vi "students-estimator.vi"() -> (0 "Estimator Script Error":errorcluster, 1 "Estimator State Space Object":T2 {"Transport Delay" format="%.2f"; "D" format="%#.2g"; "C" format="%#.2g"; "B" format="%#.2g"; "A" format="%#.2g"; "properties"."Sampling Time" format="%#.6p"; "properties"."Output Delays" format="%.4f"; "properties"."Input Delays" format="%.4f"}, 2 "State Feedback Gain (K)":T1, 3 "Input Scaling (Nbar)":dbl)   [LabVIEW 2009]
uses:
  <vilib>/addons/Control Design/_Model Construction/Model Typedefs.llb/CD State Space Model (MIMO).ctl
  <vilib>/addons/Control Design/_Model Construction/Model Typedefs.llb/CD General Elements.ctl
  <vilib>/Analysis/Matrix/Datatypes/RealMatrix.ctl
  <vilib>/imath/engines/lvmath2/RunTimeEngine/ErrorHandling/NIMS_Finalize Error.vi
  <vilib>/imath/engines/lvmath2/RunTimeEngine/Parser/MC_Version.vi
  <vilib>/imath/engines/lvmath2/RunTimeEngine/NodeEndStatement/NIMS_NodeEndStatement_Output.vi
  <instcachedir>/0/NIMS_NodeEndStatement_Output_53EC0D466D134D7ABD903AC30B43404B.lvgen/NIMS_NodeEndStatement_Output_53EC0D466D134D7ABD903AC30B43404B_004.vi
  <instcachedir>/0/NIMS_NodeEndStatement_Output_53EC0D466D134D7ABD903AC30B43404B.lvgen/NIMS_NodeEndStatement_Output_53EC0D466D134D7ABD903AC30B43404B_003.vi
  <instcachedir>/0/NIMS_NodeEndStatement_Output_53EC0D466D134D7ABD903AC30B43404B.lvgen/NIMS_NodeEndStatement_Output_53EC0D466D134D7ABD903AC30B43404B_002.vi
  <instcachedir>/0/NIMS_NodeEndStatement_Output_53EC0D466D134D7ABD903AC30B43404B.lvgen/NIMS_NodeEndStatement_Output_53EC0D466D134D7ABD903AC30B43404B_001.vi
  <instcachedir>/0/NIMS_NodeEndStatement_Output_53EC0D466D134D7ABD903AC30B43404B.lvgen/NIMS_NodeEndStatement_Output_53EC0D466D134D7ABD903AC30B43404B_000.vi
  <vilib>/imath/engines/lvmath/Functions/Error Handling/MergeErrorsWrapper.vi
  <vilib>/imath/engines/lvmath2/RunTimeEngine/NodeEndStatement/NIMS_NodeEndStatement_Get Vector.vi
  <instcachedir>/0/NIMS_NodeEndStatement_Get Vector_708AE642CFEE4B9892E482CBBBA3A4D6.lvgen/NIMS_NodeEndStatement_Get Vector_708AE642CFEE4B9892E482CBBBA3A4D6_000.vi
  <vilib>/Analysis/Matrix/Numeric/Conversions/Array To Matrix - RA2.vi
  <vilib>/imath/engines/lvmath/Plug In/Control Design/BuiltInFunctions/pzgraph/NIMS_CD_[Poles,Zeros]=pzgraph(SS).vi
  <vilib>/imath/engines/lvmath/Plug In/Control Design/BuiltInFunctions/ss/NIMS_CD_ss(A,B,C,D).vi
  <vilib>/imath/engines/lvmath/Plug In/Control Design/BuiltInFunctions/lqr/NIMS_CD_lqr(A,B,Q,R,N).vi
  <vilib>/imathl/engines/lvmath/Functions/Error Handling/Create Error.vi
  <vilib>/imath/engines/lvmath2/RunTimeEngine/ArithmeticOperatorToken/NIMS_ArithmeticOperator_plus.vi
  <instcachedir>/0/NIMS_ArithmeticOperator_plus_48B9519178ED42D7840F01273E784BFE.lvgen/NIMS_ArithmeticOperator_plus_48B9519178ED42D7840F01273E784BFE_000.vi
  <vilib>/imath/engines/lvmath2/RunTimeEngine/BuiltInFunctions/imag/NIMS_imag(Complex).vi
  <instcachedir>/0/NIMS_imag(Complex)_3180D40D00C843A49C2B33397F857BF3.lvgen/NIMS_imag(Complex)_3180D40D00C843A49C2B33397F857BF3_000.vi
  <vilib>/imath/engines/lvmath/Plug In/Control Design/BuiltInFunctions/poleplace/NIMS_CD_poleplace(A,B,poles,STR).vi
  <vilib>/imath/engines/lvmath2/RunTimeEngine/RowToken/NIMS_RowToken_M_CV.vi
  <instcachedir>/0/NIMS_RowToken_M_CV_81A7A755B26C4322943C4DA5F8800EF8.lvgen/NIMS_RowToken_M_CV_81A7A755B26C4322943C4DA5F8800EF8_000.vi
  <vilib>/imath/engines/lvmath/Functions/Error Handling/MC_Error Cluster From Error Code.vi
  <vilib>/imath/engines/lvmath2/RunTimeEngine/ArithmeticOperatorToken/NIMS_ArithmeticOperator_multmx(M,CV).vi
  <instcachedir>/0/NIMS_ArithmeticOperator_multmx(M,CV)_C209B7F61D9F434AA9A64D69928E507A.lvgen/NIMS_ArithmeticOperator_multmx(M,CV)_C209B7F61D9F434AA9A64D69928E507A_001.vi
  <vilib>/imath/engines/lvmath2/RunTimeEngine/BuiltInFunctions/inv/NIMS_inv(GM).vi
  <instcachedir>/0/NIMS_inv(GM)_A6DF8FE880224208AACFE4CF9F659502.lvgen/NIMS_inv(GM)_A6DF8FE880224208AACFE4CF9F659502_000.vi
  <vilib>/imath/engines/lvmath2/RunTimeEngine/BuiltInFunctions/zeros/NIMS_V=zeros(I32,I32).vi
  <vilib>/imath/engines/lvmath2/RunTimeEngine/BuiltInFunctions/size/NIMS_I32=size(GM,I32).vi
  <instcachedir>/0/NIMS_I32=size(GM,I32)_534EB74D584742B4AAC17727D9B9DE44.lvgen/NIMS_I32=size(GM,I32)_534EB74D584742B4AAC17727D9B9DE44_000.vi
  <vilib>/imath/engines/lvmath2/RunTimeEngine/VariableToken/Read/NIMS_Get Elements - SorM(_) - Check.vi
  <instcachedir>/0/NIMS_Get Elements - SorM(_) - Check_19F9AFF5C34A45CBABECD1A546CADF04.lvgen/NIMS_Get Elements - SorM(_) - Check_19F9AFF5C34A45CBABECD1A546CADF04_002.vi
  <vilib>/imath/engines/lvmath2/RunTimeEngine/RangeToken/NIMS_Range_R2.vi
  <instcachedir>/0/NIMS_Get Elements - SorM(_) - Check_19F9AFF5C34A45CBABECD1A546CADF04.lvgen/NIMS_Get Elements - SorM(_) - Check_19F9AFF5C34A45CBABECD1A546CADF04_000.vi
  <vilib>/imath/engines/lvmath2/RunTimeEngine/ArithmeticOperatorToken/NIMS_ArithmeticOperator_multmx(RV,M).vi
  <instcachedir>/0/NIMS_ArithmeticOperator_multmx(RV,M)_604D030E1B8D4CCEAC41A6F25BE299B2.lvgen/NIMS_ArithmeticOperator_multmx(RV,M)_604D030E1B8D4CCEAC41A6F25BE299B2_001.vi
  <vilib>/Analysis/Matrix/NI_Matrix.lvlib
  <vilib>/addons/Control Design/_Model Construction/NI_LinSys_Model Typedefs.lvlib
panel:
  out "Controller Poles":cdb[](array[numeric])
  out "Observer poles":cdb[](array[numeric])
  out "Open Loop Poles":cdb[](array[numeric])
  out "Open Loop Zeros":cdb[](array[numeric])
  out "K":dbl[](array[numeric])
  out "L":dbl[](array[numeric])
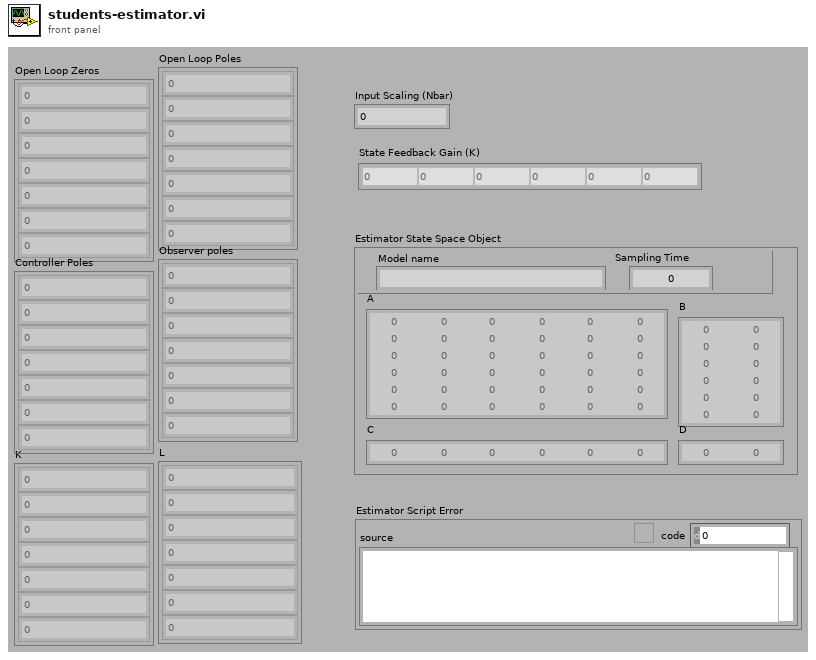
[diagram p1: front panel]
types:
  T1 = typedef "NI_Matrix.lvlib/RealMatrix.ctl" = dbl[][]
  T2 = typedef "NI_LinSys_Model Typedefs.lvlib/CD State Space Model (MIMO).ctl" = cluster{"properties":T3, "A":dbl[][], "B":dbl[][], "C":dbl[][], "D":dbl[][], "StateNames":string[], "Transport Delay":dbl[][]}
  T3 = typedef "NI_LinSys_Model Typedefs.lvlib/CD General Elements.ctl" = cluster{"Model name":string, "Input names":string[], "Output names":string[], "Input Delays":dbl[], "Output Delays":dbl[], "Sampling Time":dbl, "Notes":string}
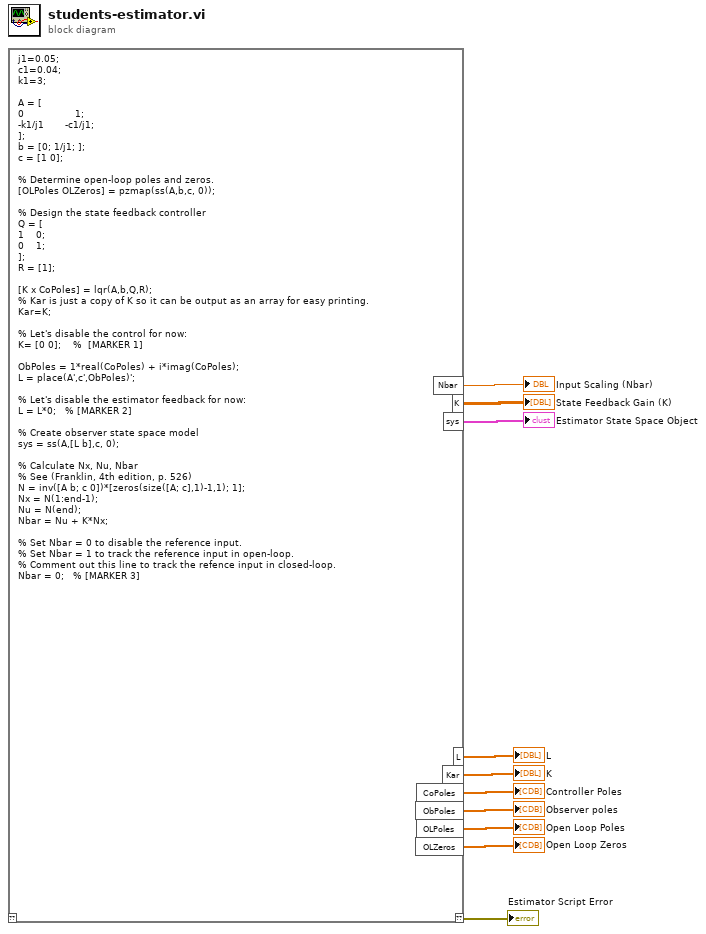
[diagram p0: block diagram]
diagram:
  n1 = mathscript code="j1=0.05;\nc1=0.04;\nk1=3;\n\nA = [\n0                 1;\n-k1/j1       -c1/j1;\n];\nb = [0; 1/j1; ];\nc = [1 0];\n\n% Determine open-loop poles and zeros.\n[OLPoles OLZeros] = pzmap(ss(A,b,c, 0));\n\n% Design the state feedback controller\nQ = [\n1    0;\n0    1;\n];\nR = [1];\n\n[K x CoPoles] = lqr(A,b,Q,R);\n% Kar is just a copy of K so it can be output as an array for easy printing.\nKar=K;\n\n% Let's disable the control for now:\nK= [0 0];    %  [MARKER 1]\n\nObPoles = 1*real(CoPoles) + i*imag(CoPoles);\nL = place(A',c',ObPoles)';\n\n% Let's disable the estimator feedback for now:\nL = L*0;   % [MARKER 2]\n\n% Create observer state space model\nsys = ss(A,[L b],c, 0);\n\n% Calculate Nx, Nu, Nbar \n% See (Franklin, 4th edition, p. 526)\nN = inv([A b; c 0])*[zeros(size([A; c],1)-1,1); 1];\nNx = N(1:end-1);\nNu = N(end);\nNbar = Nu + K*Nx;\n\n% Set Nbar = 0 to disable the reference input.\n% Set Nbar = 1 to track the reference input in open-loop.\n% Comment out this line to track the refence input in closed-loop.\nNbar = 0;   % [MARKER 3]"() -> ("??"=→"Estimator Script Error":errorcluster, "sys"=→"Estimator State Space Object":T2, "K"=→"State Feedback Gain (K)":T1, "Nbar"=→"Input Scaling (Nbar)":dbl, "L"=→"L":dbl[], "Kar"=→"K":dbl[], "OLPoles"=→"Open Loop Poles":cdb[], "OLZeros"=→"Open Loop Zeros":cdb[], "ObPoles"=→"Observer poles":cdb[], "CoPoles"=→"Controller Poles":cdb[])  [unwired: 1 in]
